vi "ex6_trigger_color.vi"() -> ()   [LabVIEW 2012]
uses:
  \\csehomes\csehome$/dsp15/My Documents/Mini-Cryo Automation Software/Patiwet/QCam.llb/QCam Grab Abort.vi
panel:
  in  "Halt loop":bool
  in  "Trigger Mode":T1(ring)=enum."Edge hi"
  in  "stop":bool
  out "error status":errorcluster
  out "Preview Window":picture
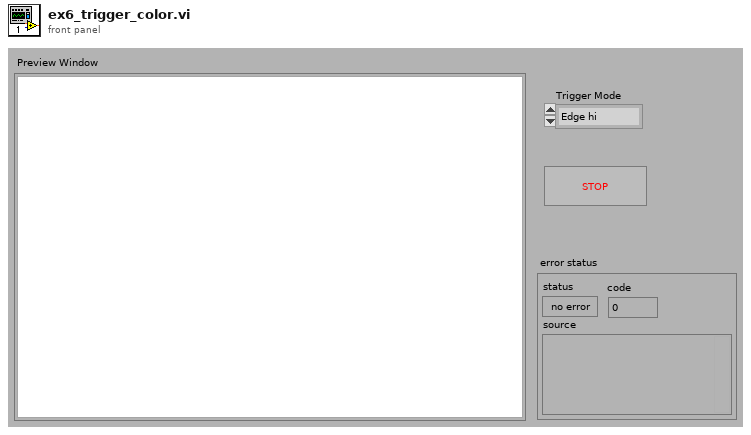
[diagram p1: front panel]
types:
  T1 = enum32{"Freerun", "Edge hi", "Edge low", "Pulse hi", "Pulse low", "Software"}
  T2 = typedef "Image Type" = u32
  T3 = typedef "IMAQ Image.ctl" = refnum<image>
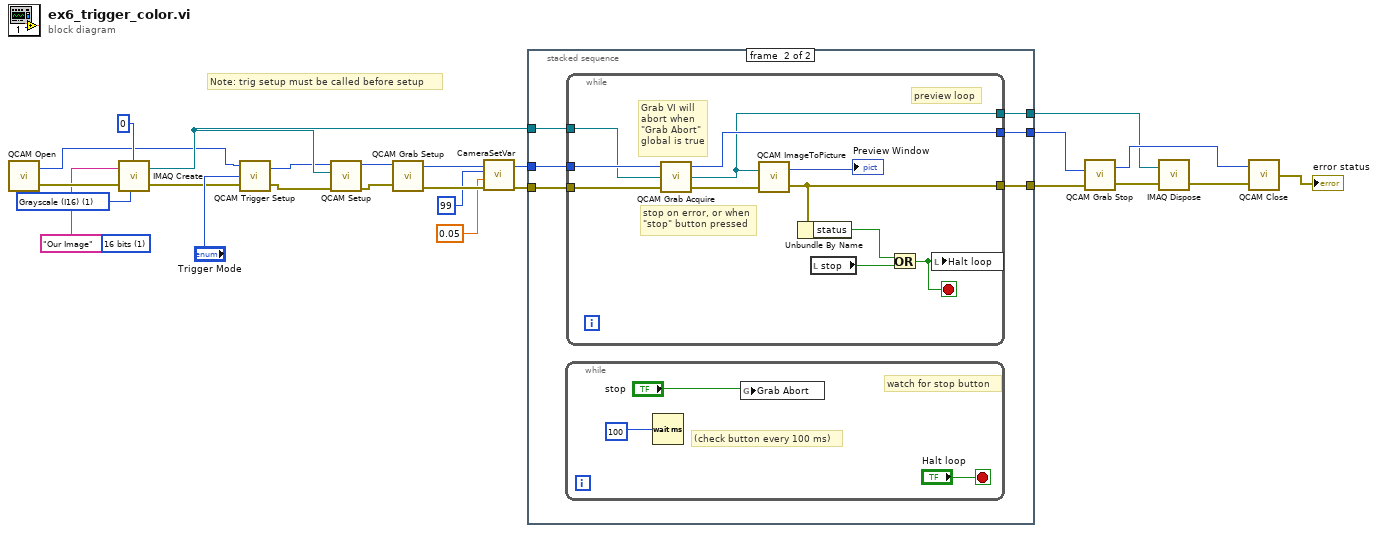
[diagram p0: block diagram]
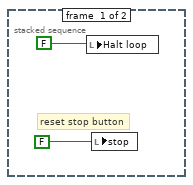
[diagram p2: hidden frame]
diagram:
  w1 = T2 1 items=["Grayscale (U8)", "Grayscale (I16)", "Grayscale (SGL)", "Complex (CSG)", "RGB (U32)", "HSL (U32)", "RGB (U64)", "Grayscale (U16)"] ("Image Type")
  (unwired) u32 1 items=["8 bits", "16 bits"] ("Image Type")
  # "Note: trig setup must be called before setup"
  n1 = call "QCAM Open.vi"() -> ("error out"=w24:errorcluster, "cameraId out"=w5:u32)  [unwired: 2 in]
  n2 = call "IMAQ Create"("Border Size"=0, "Image Name"="Our Image", "Image Type"=w1, "error in (no error)"=w24) -> ("New Image"=w18:T3, "error out"=w8:errorcluster)  [unwired: 1 out]
  n3 = call "QCAM Trigger Setup.vi"("error in (no error)"=w8, "trigger mode"="Trigger Mode", "camera Id"=w5) -> ("error out"=w7:errorcluster, "camera Id out"=w6:u32)
  n4 = call "QCAM Setup.vi"("error in (no error)"=w7, "Image"=w18, "cameraId"=w6) -> ("error out"=w10:errorcluster, "cameraId out"=w9:u32)  [unwired: 3 in, 4 out]
  n5 = call "QCAM Grab Setup.vi"("error in (no error)"=w10, "cameraId"=w9) -> ("error out"=w20:errorcluster, "cameraId out"=w19:u32)
  n6 = call <userlib>:"CameraSetVar.vi"("error in"=w20, "Value"=0.05, "Parameter ID"=99) -> ("error out"=w4:errorcluster)  [unwired: 1 in, 1 out]
  n7 = stacked-sequence {
    tunnel: w4 -> [_ w32]
    tunnel: w19 -> [_ w31]
    tunnel: w18 -> [_ w30]
    tunnel: [_ w29] -> w17
    tunnel: [_ w28] -> w16
    tunnel: [_ w27] -> w13
    frame #0 {
      # "reset stop button"
      n8 = local write "Halt loop"(FALSE) -> ()
      n9 = local write "stop"(FALSE) -> ()
    }
    frame #1 {
      n10 = while {
        stop <- "Halt loop" stop-if-true
        # "(check button every 100 ms)"
        # "watch for stop button"
        n11 = Wait (ms)(milliseconds to wait=100) -> ()  [unwired: 1 out]
        n12 = global write "QCam Grab Abort.vi" "Grab Abort"("stop") -> ()
      }
      n13 = while {
        tunnel: [w38] -> w27
        tunnel: [w35] -> w29
        tunnel: w30 -> [w36]
        tunnel: w31 -> [w37]
        tunnel: w32 -> [w40]
        tunnel: [w41] -> w28
        stop <- w33 stop-if-true
        # "Grab VI will abort when \"Grab Abort\" global is true"
        # "preview loop"
        # "stop on error, or when \"stop\" button pressed"
        n14 = call "QCAM Grab Acquire.vi"("error in (no error)"=w40, "Image"=w36, "cameraId"=w37) -> ("error out"=w42:errorcluster, "Image Out"=w38:T3, "cameraId out"=w41:u32)
        n15 = call <userlib>:"QCAM ImageToPicture.vi"("error in (no error)"=w42, "Image"=w38) -> ("error out"=w35:errorcluster, "Picture Out"=→"Preview Window":picture)
        n16 = Unbundle By Name(w35) -> ("status"=w39:bool)
        n17 = local read "stop"() -> (w34:bool)
        n18 = Or(x=w39, y=w34) -> (x .or. y?=w33:bool)
        n19 = local write "Halt loop"(w33) -> ()
      }
    }
  }
  n20 = call "QCAM Grab Stop.vi"("error in (no error)"=w17, "cameraId"=w16) -> ("error out"=w23:errorcluster, "cameraId Out"=w21:u32)
  n21 = call "IMAQ Dispose"("Image"=w13, "error in (no error)"=w23) -> ("error out"=w22:errorcluster)  [unwired: 1 in, 3 out]
  n22 = call "QCAM Close.vi"("error in (no error)"=w22, "cameraId"=w21) -> ("error out"=→"error status":errorcluster)
